vi "Open.vi"(8 "error in (no error)":errorcluster, 11 "VISA resource name":refnum<visa-resource-name>) -> (0 "error out":errorcluster, 3 "GE 5565PIORC.lvclass":refnum<class "GE 5565PIORC.lvclass">)   [LabVIEW 2016, in "GE 5565PIORC.lvclass"]
uses:
  GE 5565PIORC.lvclass
  GE 5565PIORC/GE 5565PIORC Old.lvclass
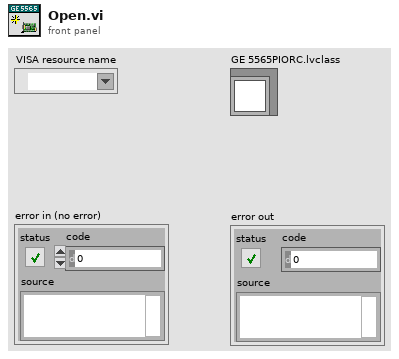
[diagram p1: front panel]
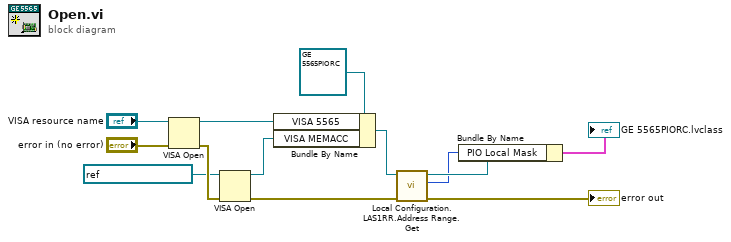
[diagram p0: block diagram]
diagram:
  n1 = VISA Open(error in (no error)="error in (no error)", VISA resource name="VISA resource name") -> (VISA resource name=w13:refnum<visa-resource-name>, error out=w12:errorcluster)  [unwired: 3 in]
  n2 = VISA Open(error in (no error)=w12, VISA resource name=refnum<visa-resource-name> "PXI0::MEMACC") -> (VISA resource name=w10:refnum<visa-resource-name>, error out=w9:errorcluster)  [unwired: 3 in]
  n3 = Bundle By Name(cluster=refnum<class "GE 5565PIORC.lvclass"> refnum ("GE 5565PIORC.lvclass"), "VISA 5565"=w13, "VISA MEMACC"=w10) -> (w8:refnum<class "GE 5565PIORC.lvclass">)
  n4 = call "Local Configuration.LAS1RR.Address Range.Get.vi"("error in (no error)"=w9, "GE 5565PIORC"=w8) -> ("error out"=→"error out":errorcluster, "Address Range"=w6:u32, "GE 5565PIORC out"=w7:refnum<class "GE 5565PIORC Old.lvclass">)  [unwired: 7 in]
  n5 = Bundle By Name(cluster=w7, "PIO Local Mask"=w6) -> (→"GE 5565PIORC.lvclass":cluster{})
